vi "Mag_&_Temp_Cntrl.vi"() -> ()   [LabVIEW 2025]
uses:
  CTLS/Status Indicators.ctl
  CTLS/Sweeper.ctl
  CTLS/Scan_Params (QMH).ctl
  CTLS/PSU Status.ctl
  CTLS/TC-Cluster.ctl
  CTLS/ACK.ctl
  <userlib>/Nanonis Prog Interface V5e/Nanonis Prog Interface.lvlib
panel:
  in  "Field and Temp Array Controller":cluster{"Field (T)":dbl[], "Temps (K)":dbl[]}
  out "Status Indicator":T1={"Sweep States"=enum."1. Idle", "PointStep"=enum."1. Scan_1", "Current Field"=0.0, "Current Temp"=0.0, "Expected_ACK"=enum."1. None", "AfterAckStep"=enum."1. Idle", "Current Index Field"=0, "Current Index Temp"=0, "ACK Structure "=enum."Inner"}
  in  "Stop Button":bool
  in  "Stop Experiment":bool
  in  "Start Experiment":bool
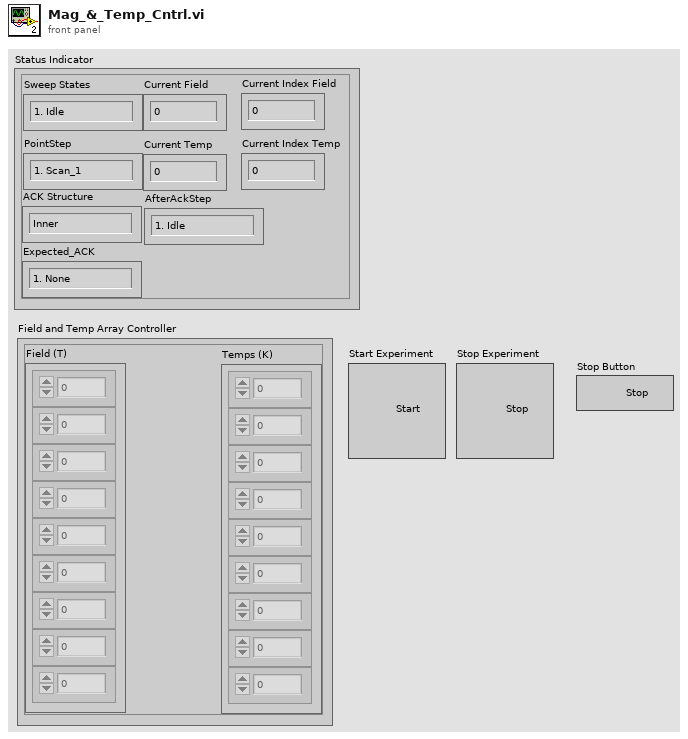
[diagram p1: front panel]
types:
  T1 = typedef "Status Indicators.ctl" = cluster{"Sweep States":enum16{"1. Idle", "2. Start", "3. Apply_Config", "4. Run_Point_Step", "5. Wait ACK", "6. Next Field", "7. Next Temp", "8. Stop"}, "PointStep":enum16{"1. Init_Bias", "2. Init_Scan", "3. Field_Stable", "4. Temp_stable", "1. Scan_1", "2. DC_SF_1", "3. DC_BS_1", "4. Bias", "5. Scan_2", "6. DC_SF_2", "7. DC_BS_2", "8. Done"}, "Current Field":dbl, "Current Temp":dbl, "Expected_ACK":enum16{"1. None", "2. TempStable", "3. FieldStable", "4. ConfigApplied", "5. ScanDone", "6. BiasDone", "7. DriftDone (SF)", "8. DrifDone (BS)", "9. Done"}, "AfterAckStep":enum16{"1. Idle", "2. Start", "3. Apply_Config", "4. Run_Point_Step", "5. Wait ACK", "6. Next Field", "7. Next Temp", "8. Stop"}, "Current Index Field":i32, "Current Index Temp":i32, "ACK Structure ":enum16{"Inner", "Outer"}}
  T2 = enum16{"1. INIT TEMP", "2. TC ON", "3. TEMP_STAB", "4. TC IDLE", "5. TC OFF (Reset)"}
  T3 = typedef "TC-Cluster.ctl" = cluster{"Range (0:Off)":u16, "Manual Output (0.00 %)":dbl, "Rate (D) (0.0 %)":dbl, "Reset (I) (20.0)":dbl, "Gain (P) (50.0)":dbl, "Power Up Enable (F: Disable)":bool, "Max User Current (2.000)":dbl, "Heater Resistance (1:25 Ohms)":u16, "Max Current (0:User Specified)":u16, "Heater Out Display (1:Current)":u16, "Mode (0:Off)":u16, "Input (0:None)":u16, "Target Temp (K)":dbl, "Serial Configuration":cluster{"Baud Rate":u32, "Parity":u16, "Data Bits":u16, "Stop Bits":u16, "Flow Control":u16}, "VISA resource name":refnum<visa-resource-name>, "Configure Control Parameters (0: Configure)":u16, "Enable Setpoint (F:Disable)":bool, "Input (0:A)":u16, "Data Source (0:Kelvin)":u16, "Output's Control Loop (1:1)":u16, "STND DEV Threshold ":dbl, "Mean Tolerance ":dbl, "Current State":enum16{"1. INIT TEMP", "2. TC ON", "3. TEMP_STAB", "4. TC IDLE", "5. TC OFF (Reset)"}}
  T4 = enum16{"1. Idle", "2. Start", "3. Apply_Config", "4. Run_Point_Step", "5. Wait ACK", "6. Next Field", "7. Next Temp", "8. Stop"}
  T5 = typedef "Sweeper.ctl" = cluster{"Temps(K)":dbl[], "Fields(T)":dbl[], "Sweep States":enum16{"1. Idle", "2. Start", "3. Apply_Config", "4. Run_Point_Step", "5. Wait ACK", "6. Next Field", "7. Next Temp", "8. Stop"}, "PointStep":enum16{"1. Init_Bias", "2. Init_Scan", "3. Field_Stable", "4. Temp_stable", "1. Scan_1", "2. DC_SF_1", "3. DC_BS_1", "4. Bias", "5. Scan_2", "6. DC_SF_2", "7. DC_BS_2", "8. Done"}, "Current Field":dbl, "Current Temp":dbl, "Expected_ACK":enum16{"1. None", "2. TempStable", "3. FieldStable", "4. ConfigApplied", "5. ScanDone", "6. BiasDone", "7. DriftDone (SF)", "8. DrifDone (BS)", "9. Done"}, "ACK":enum16{"1. None", "2. TempStable", "3. FieldStable", "4. ConfigApplied", "5. ScanDone", "6. BiasDone", "7. DriftDone (SF)", "8. DrifDone (BS)", "9. Done"}, "AfterAckStep":enum16{"1. Idle", "2. Start", "3. Apply_Config", "4. Run_Point_Step", "5. Wait ACK", "6. Next Field", "7. Next Temp", "8. Stop"}, "Current Index Field":i32, "Current Index Temp":i32, "ACK Structure ":enum16{"Inner", "Outer"}}
  T6 = enum16{"1. INIT MAG", "2. MAG ON", "3. MAG_STAB", "4. MAG IDLE", "5. MAG OFF (Reset)"}
  T7 = typedef "PSU Status.ctl" = cluster{"Ramp Target":enum16{"ZERO", "MID", "MAX"}, "Pause":bool, "Switch Heater":bool, "Persistent Field":dbl, "Persistent Current":dbl, "Tesla":bool, "Output (T)":dbl, "Output (A)":dbl, "X Trip":enum16{"DISABLED", "ENABLED", "ACTIVE"}, "Ramp Rate (A/s)":dbl, "V Limit (V)":dbl, "Heater Voltage":dbl, "MAX Setpoint (A)":dbl, "MAX Setpoint (T)":dbl, "MID Setpoint (A)":dbl, "MID Setpoint (T)":dbl, "Lock":bool, "Field Constant":dbl, "Remote":bool, "Direction":enum16{"POSITIVE", "NEGATIVE", "OPEN", "UNIPOLAR"}, "Helium Level":u16, "Quench !":bool, "Voltage":dbl, "V Limit !":bool, "Ramping":bool, "At Target":bool, "Trip Field":dbl, "Trip Current":dbl, "Current State":enum16{"1. INIT MAG", "2. MAG ON", "3. MAG_STAB", "4. MAG IDLE", "5. MAG OFF (Reset)"}, "MAG Reference":refnum<visa-resource-name>}
  T8 = enum16{"1. BIAS", "2. POLL BIAS", "3. SCAN", "4. SCAN_IDLE", "5. Drift_Correct (SF)", "6. Drift_Correct (BS)", "7. STOP"}
  T9 = typedef "Scan_Params (QMH).ctl" = cluster{"Setpoint (I)":dbl[], "Bias (V)":dbl[], "Number of scans":u8, "Port number (3364)":u32, "Avoid zero threshold (V)":dbl, "Current State":enum16{"1. BIAS", "2. POLL BIAS", "3. SCAN", "4. SCAN_IDLE", "5. Drift_Correct (SF)", "6. Drift_Correct (BS)", "7. STOP"}}
  T10 = typedef "ACK.ctl" = cluster{"ACK":enum16{"1. None", "2. TempStable", "3. FieldStable", "4. ConfigApplied", "5. ScanDone", "6. BiasDone", "7. DriftDone (SF)", "8. DrifDone (BS)"}}
  T11 = enum16{"1. None", "2. TempStable", "3. FieldStable", "4. ConfigApplied", "5. ScanDone", "6. BiasDone", "7. DriftDone (SF)", "8. DrifDone (BS)"}
  T12 = enum16{"1. Init_Bias", "2. Init_Scan", "3. Field_Stable", "4. Temp_stable", "1. Scan_1", "2. DC_SF_1", "3. DC_BS_1", "4. Bias", "5. Scan_2", "6. DC_SF_2", "7. DC_BS_2", "8. Done"}
  T13 = enum16{"1. None", "2. TempStable", "3. FieldStable", "4. ConfigApplied", "5. ScanDone", "6. BiasDone", "7. DriftDone (SF)", "8. DrifDone (BS)", "9. Done"}
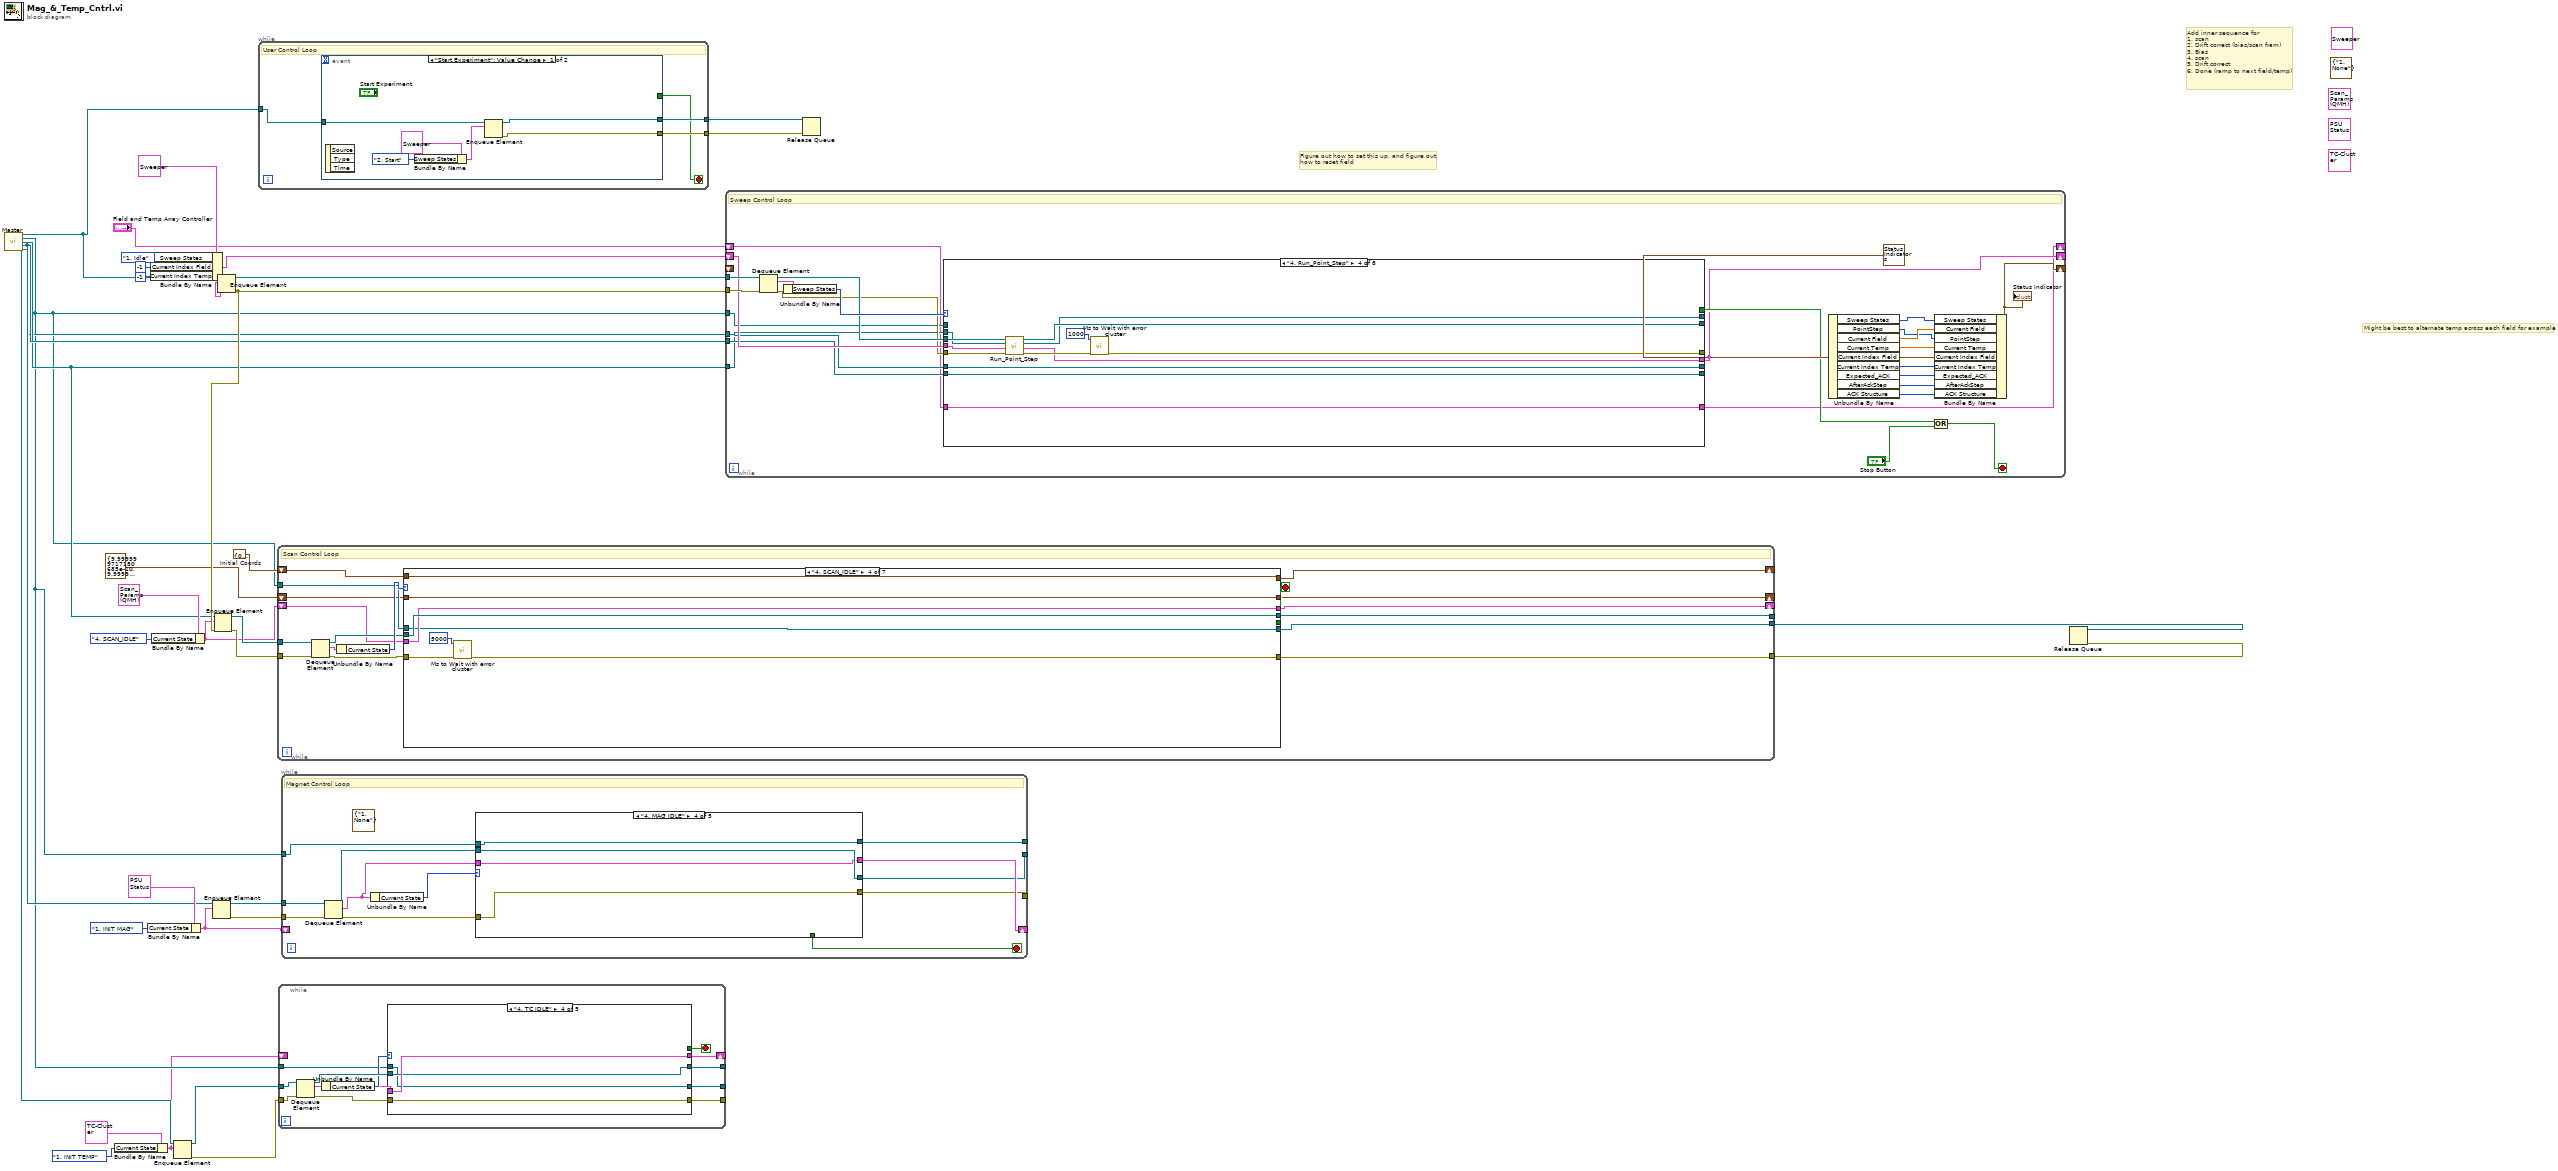
[diagram p0: block diagram]
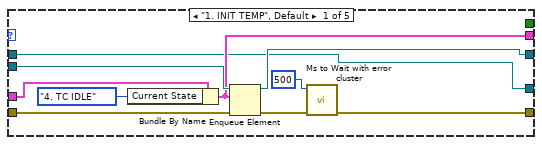
[diagram p2: hidden frame]
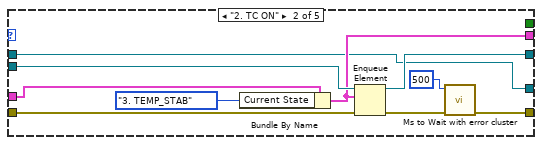
[diagram p3: hidden frame]
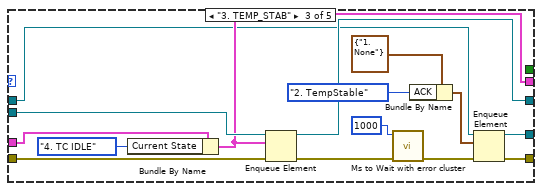
[diagram p4: hidden frame]
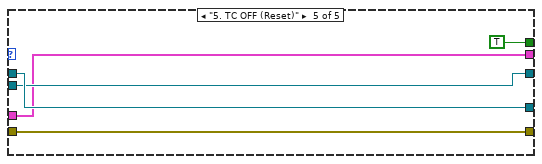
[diagram p5: hidden frame]
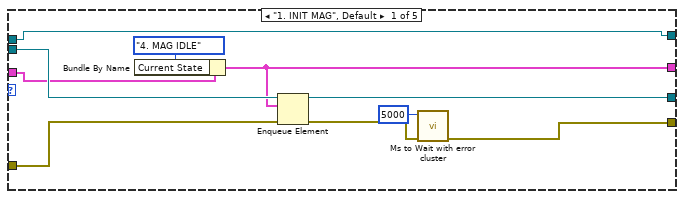
[diagram p6: hidden frame]
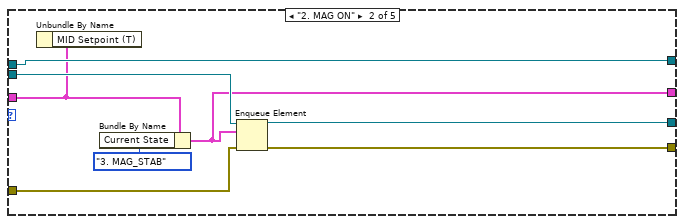
[diagram p7: hidden frame]
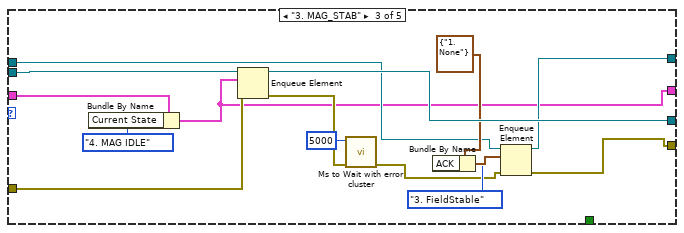
[diagram p8: hidden frame]
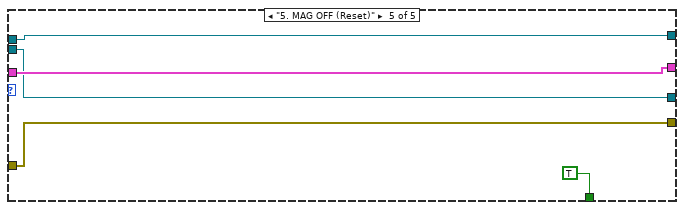
[diagram p9: hidden frame]
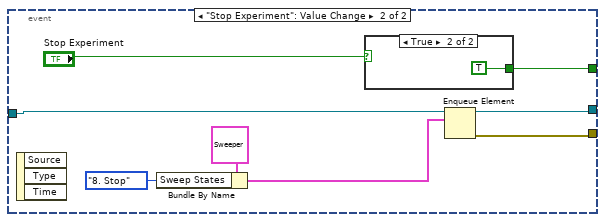
[diagram p10: hidden frame]
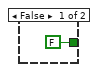
[diagram p11: hidden frame]
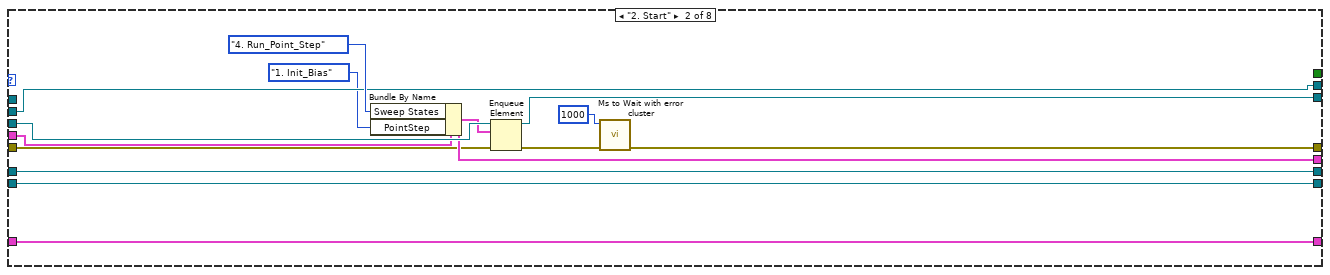
[diagram p13: hidden frame]
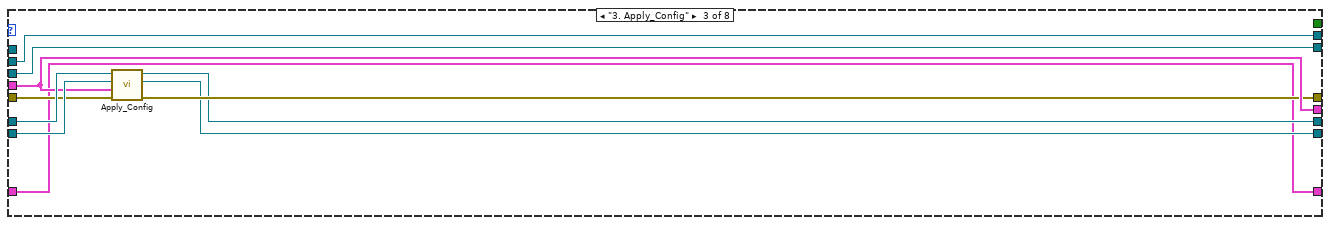
[diagram p14: hidden frame]
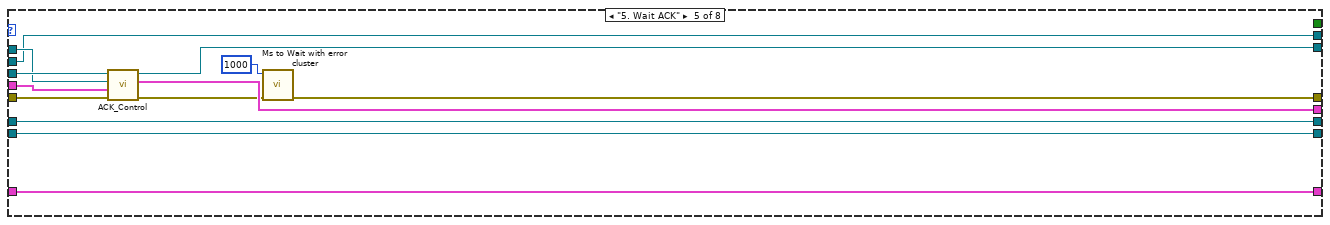
[diagram p15: hidden frame]
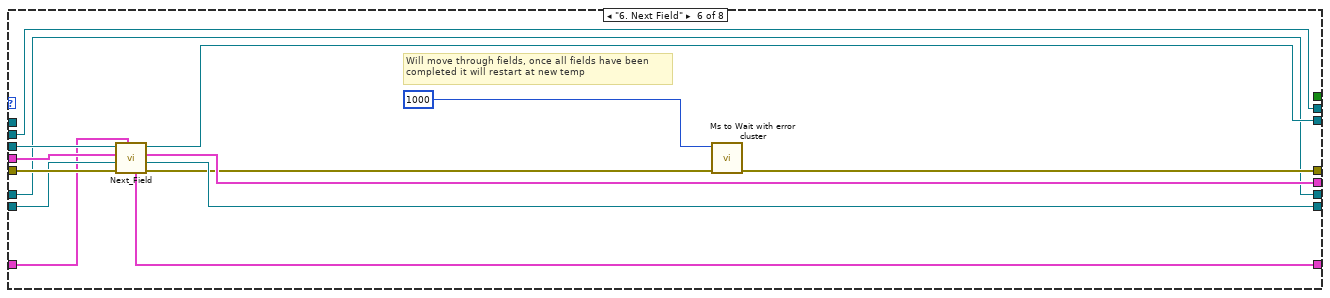
[diagram p16: hidden frame]
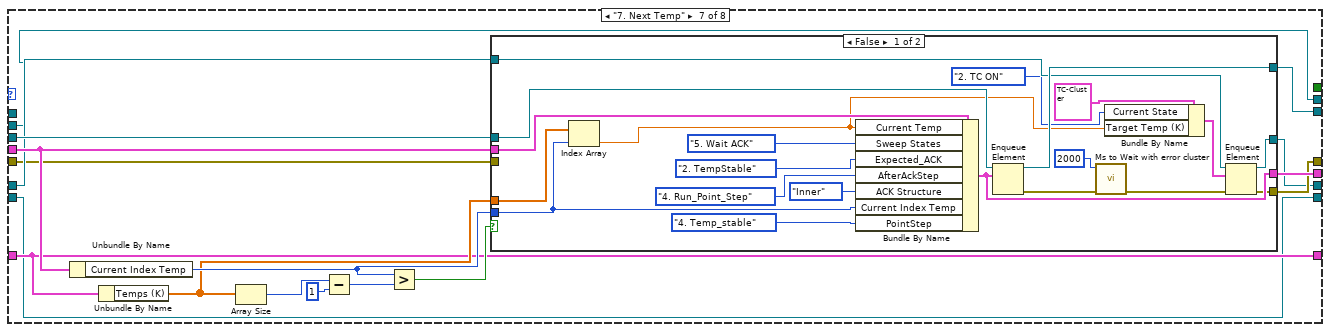
[diagram p17: hidden frame]
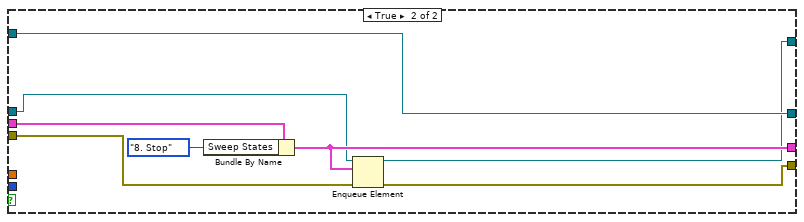
[diagram p18: hidden frame]
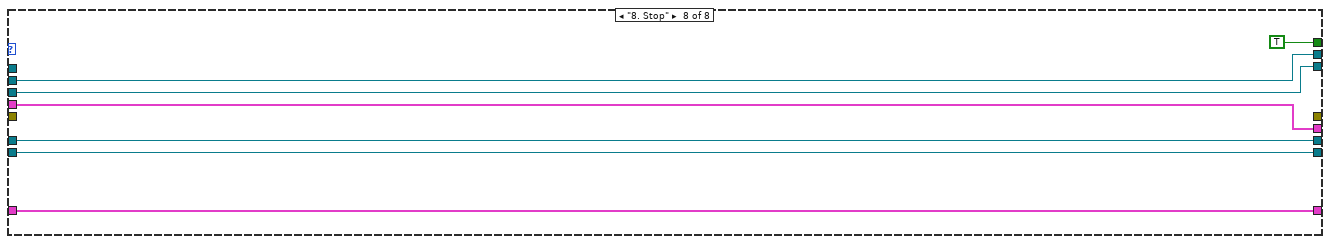
[diagram p19: hidden frame]
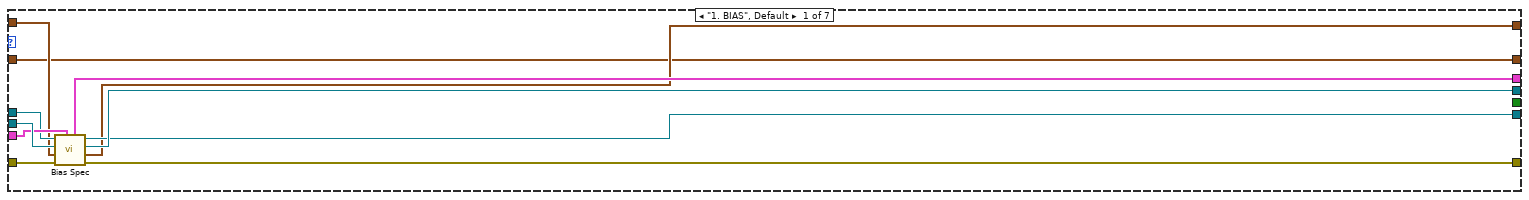
[diagram p20: hidden frame]
diagram:
  w15 = cluster{"Initial x":dbl, "Initial y":dbl} {"Initial x"=0.0, "Initial y"=0.0}  # Initial Coords
  (unwired) T10 {"ACK"=enum."1. None"} ("Acknowledements")
  (unwired) T5 {"Temps(K)"=[], "Fields(T)"=[], "Sweep States"=enum."1. Idle", "PointStep"=enum."1. Scan_1", "Current Field"=0.0, "Current Temp"=0.0, "Expected_ACK"=enum."1. None", "ACK"=enum."1. None", "AfterAckStep"=enum."1. Idle", "Current Index Field"=0, "Current Index Temp"=0, "ACK Structure "=enum."Inner"} ("Temp and Field Range")
  (unwired) T3 {"Range (0:Off)"=0, "Manual Output (0.00 %)"=0.0, "Rate (D) (0.0 %)"=0.0, "Reset (I) (20.0)"=20.0, "Gain (P) (50.0)"=50.0, "Power Up Enable (F: Disable)"=FALSE, "Max User Current (2.000)"=2.0, "Heater Resistance (1:25 Ohms)"=1, "Max Current (0:User Specified)"=0, "Heater Out Display (1:Current)"=1, "Mode (0:Off)"=0, "Input (0:None)"=0, "Target Temp (K)"=0.0, "Serial Configuration"={"Baud Rate"=57600, "Parity"=1, "Data Bits"=7, "Stop Bits"=10, "Flow Control"=0}, "VISA resource name"="", "Configure Control Parameters (0: Configure)"=0, "Enable Setpoint (F:Disable)"=FALSE, "Input (0:A)"=0, "Data Source (0:Kelvin)"=0, "Output's Control Loop (1:1)"=1, "STND DEV Threshold "=0.1, "Mean Tolerance "=0.02, "Current State"=enum."1. INIT TEMP"} ("Temp Controller")
  (unwired) T9 {"Setpoint (I)"=[], "Bias (V)"=[], "Number of scans"=1, "Port number (3364)"=3364, "Avoid zero threshold (V)"=0.004999999888241291, "Current State"=enum."1. BIAS"} ("Scan Parameters")
  (unwired) T7 {"Ramp Target"=enum."ZERO", "Pause"=FALSE, "Switch Heater"=FALSE, "Persistent Field"=0.0, "Persistent Current"=0.0, "Tesla"=FALSE, "Output (T)"=0.0, "Output (A)"=0.0, "X Trip"=enum."DISABLED", "Ramp Rate (A/s)"=0.0, "V Limit (V)"=0.0, "Heater Voltage"=0.0, "MAX Setpoint (A)"=0.0, "MAX Setpoint (T)"=0.0, "MID Setpoint (A)"=0.0, "MID Setpoint (T)"=0.0, "Lock"=FALSE, "Field Constant"=0.0, "Remote"=FALSE, "Direction"=enum."POSITIVE", "Helium Level"=0, "Quench !"=FALSE, "Voltage"=0.0, "V Limit !"=FALSE, "Ramping"=FALSE, "At Target"=FALSE, "Trip Field"=0.0, "Trip Current"=0.0, "Current State"=enum."1. INIT MAG", "MAG Reference"="COM4"} ("PSU Status In")
  # "Figure out how to set this up, and figure out\nhow to reset field"
  # "Might be best to alternate temp across each field for example"
  # "Add inner sequence for \n1. scan\n2. Drift correct (bias/scan fram)\n3. Bias\n4. scan\n5. Drift correct\n6. Done (ramp to next field/temp)"
  n1 = call "Master.vi"() -> ("SweepQ"=w32:refnum<queue>, "ACK Q"=w3:refnum<queue>, "ScanQ"=w12:refnum<queue>, "MagQ"=w13:refnum<queue>, "TempQ"=w8:refnum<queue>)  [unwired: 11 in]
  n2 = Bundle By Name(cluster=T3 {"Range (0:Off)"=0, "Manual Output (0.00 %)"=0.0, "Rate (D) (0.0 %)"=0.0, "Reset (I) (20.0)"=20.0, "Gain (P) (50.0)"=50.0, "Power Up Enable (F: Disable)"=FALSE, "Max User Current (2.000)"=2.0, "Heater Resistance (1:25 Ohms)"=1, "Max Current (0:User Specified)"=0, "Heater Out Display (1:Current)"=1, "Mode (0:Off)"=0, "Input (0:None)"=0, "Target Temp (K)"=0.0, "Serial Configuration"={"Baud Rate"=57600, "Parity"=1, "Data Bits"=7, "Stop Bits"=10, "Flow Control"=0}, "VISA resource name"="", "Configure Control Parameters (0: Configure)"=0, "Enable Setpoint (F:Disable)"=FALSE, "Input (0:A)"=0, "Data Source (0:Kelvin)"=0, "Output's Control Loop (1:1)"=1, "STND DEV Threshold "=0.1, "Mean Tolerance "=0.02, "Current State"=enum."1. INIT TEMP"} ("Temp Controller"), "Current State"=T2."1. INIT TEMP") -> (w2:T3)
  n3 = Bundle By Name(cluster=T7 {"Ramp Target"=enum."ZERO", "Pause"=FALSE, "Switch Heater"=FALSE, "Persistent Field"=0.0, "Persistent Current"=0.0, "Tesla"=FALSE, "Output (T)"=0.0, "Output (A)"=0.0, "X Trip"=enum."DISABLED", "Ramp Rate (A/s)"=0.0, "V Limit (V)"=0.0, "Heater Voltage"=0.0, "MAX Setpoint (A)"=0.0, "MAX Setpoint (T)"=0.0, "MID Setpoint (A)"=0.0, "MID Setpoint (T)"=0.0, "Lock"=FALSE, "Field Constant"=0.0, "Remote"=FALSE, "Direction"=enum."POSITIVE", "Helium Level"=0, "Quench !"=FALSE, "Voltage"=0.0, "V Limit !"=FALSE, "Ramping"=FALSE, "At Target"=FALSE, "Trip Field"=0.0, "Trip Current"=0.0, "Current State"=enum."1. INIT MAG", "MAG Reference"="COM4"} ("PSU Status In"), "Current State"=T6."1. INIT MAG") -> (w19:T7)
  n4 = Bundle By Name(cluster=T5 {"Temps(K)"=[0.0, 1.0], "Fields(T)"=[0.0, 1.0], "Sweep States"=enum."1. Idle", "PointStep"=enum."1. Scan_1", "Current Field"=0.0, "Current Temp"=0.0, "Expected_ACK"=enum."1. None", "ACK"=enum."1. None", "AfterAckStep"=enum."1. Idle", "Current Index Field"=0, "Current Index Temp"=0, "ACK Structure "=enum."Inner"} ("Temp and Field Range"), "Sweep States"=T4."1. Idle", "Current Index Field"=-1, "Current Index Temp"=-1) -> (w14:T5)
  n5 = Bundle By Name(cluster=T9 {"Setpoint (I)"=[], "Bias (V)"=[], "Number of scans"=1, "Port number (3364)"=3364, "Avoid zero threshold (V)"=0.004999999888241291, "Current State"=enum."1. BIAS"} ("Scan Parameters"), "Current State"=T8."4. SCAN_IDLE") -> (w24:T9)
  n6 = Enqueue Element(queue=w8, element=w2) -> (queue out=w5:refnum<queue>, error out=w4:errorcluster)  [unwired: 2 in, 1 out]
  n7 = Enqueue Element(queue=w13, element=w19) -> (queue out=w23:refnum<queue>, error out=w22:errorcluster)  [unwired: 2 in, 1 out]
  n8 = Enqueue Element(queue=w32, element=w14) -> (queue out=w34:refnum<queue>, error out=w27:errorcluster)  [unwired: 2 in, 1 out]
  n9 = Enqueue Element(queue=w12, element=w24, error in (no error)=w27) -> (queue out=w33:refnum<queue>, error out=w28:errorcluster)  [unwired: 1 in, 1 out]
  n10 = while {
    tunnel: w32 -> [w38]
    tunnel: [w37] -> w31
    tunnel: [w36] -> w30
    stop <- w35 stop-if-true
    # "User Control Loop"
    n11 = event shown="[0] \"Start Experiment\": Value Change" {
      selector: _ -> [_ _]
      dyn-events: _ -> [_ _]
      timeout: _ -> [_ _]
      tunnel: w38 -> [w44 w52]
      tunnel: [w41 w49] -> w37
      tunnel: [w40 w48] -> w36
      tunnel: [_ w46] -> w35
      event "Start Experiment": Value Change {
        n12 = event-data() -> ()  [unwired: 1 in, 3 out]
        n13 = Bundle By Name(cluster=T5 {"Temps(K)"=[], "Fields(T)"=[], "Sweep States"=enum."1. Idle", "PointStep"=enum."1. Scan_1", "Current Field"=0.0, "Current Temp"=0.0, "Expected_ACK"=enum."1. None", "ACK"=enum."1. None", "AfterAckStep"=enum."1. Idle", "Current Index Field"=0, "Current Index Temp"=0, "ACK Structure "=enum."Inner"} ("Temp and Field Range"), "Sweep States"=T4."2. Start") -> (w42:T5)
        n14 = Enqueue Element(queue=w44, element=w42) -> (queue out=w41:refnum<queue>, error out=w40:errorcluster)  [unwired: 2 in, 1 out]
      }
      event "Stop Experiment": Value Change {
        n15 = event-data() -> ()  [unwired: 1 in, 3 out]
        n16 = Bundle By Name(cluster=T5 {"Temps(K)"=[], "Fields(T)"=[], "Sweep States"=enum."1. Idle", "PointStep"=enum."1. Scan_1", "Current Field"=0.0, "Current Temp"=0.0, "Expected_ACK"=enum."1. None", "ACK"=enum."1. None", "AfterAckStep"=enum."1. Idle", "Current Index Field"=0, "Current Index Temp"=0, "ACK Structure "=enum."Inner"} ("Temp and Field Range"), "Sweep States"=T4."8. Stop") -> (w50:T5)
        n17 = case shown="True" "Stop Experiment" {
          tunnel: [FALSE TRUE] -> w46
          frame False {
          }
          frame True {
          }
        }
        n18 = Enqueue Element(queue=w52, element=w50) -> (queue out=w49:refnum<queue>, error out=w48:errorcluster)  [unwired: 2 in, 1 out]
      }
    }
  }
  n19 = while {
    tunnel: w3 -> [w63]
    tunnel: w33 -> [w71]
    tunnel: w28 -> [w68]
    shift-right: [w60] -> _
    shift-left: w24 -> [w61]
    tunnel: [w66] -> _
    tunnel: [w64] -> w9
    tunnel: [w62] -> w10
    shift-right: [w57] -> _
    shift-left: w15 -> [w58]
    shift-right: [w55] -> _
    shift-left: cluster{"Dx":sgl, "Dy":sgl} {"Dx"=1e-09, "Dy"=1e-09} ("Dx, Dy") -> [w56]
    stop <- w59 stop-if-true
    # "Scan Control Loop"
    n20 = Dequeue Element(queue=w71, error in (no error)=w68) -> (queue out=w67:refnum<queue>, element=w70:T9, error out=w65:errorcluster)  [unwired: 1 in, 1 out]
    n21 = Unbundle By Name(w70) -> ("Current State"=w69:T8)
    n22 = case shown="\"4. SCAN_IDLE\"" w69 {
      tunnel: w67 -> [w82 w92 w102 w118 w126 w144 w162]
      tunnel: [w81 w91 w105 w118 w127 w146 w163] -> w66
      tunnel: w65 -> [w73 w90 _ w113 _ w143 _]
      tunnel: [w76 w85 w97 w116 w122 w138 w156] -> w64
      tunnel: w63 -> [w77 w89 w103 w114 w125 w145 w161]
      tunnel: [w78 w88 w104 w114 w128 w147 w164] -> w62
      tunnel: [w79 w86 w100 w117 w123 w140 w159] -> w60
      tunnel: w61 -> [w80 w87 w101 w117 w124 w141 w160]
      tunnel: [_ _ _ _ _ _ TRUE] -> w59
      tunnel: w58 -> [w75 w84 w94 w112 w119 w133 w153]
      tunnel: [w74 w84 w94 w112 w119 w130 w153] -> w57
      tunnel: w56 -> [w72 w83 w93 w111 w121 w136 w152]
      tunnel: [w72 w83 w93 w111 w120 w136 w152] -> w55
      frame "1. BIAS", Default {
        n23 = call "Bias Spec.vi"("Scan Parameters in"=w80, "error in (no error)"=w73, "Cluster"=w75, "ScanQ in"=w82, "Queue in"=w77) -> ("error out"=w76:errorcluster, "output cluster"=w74:cluster{"Initial x":dbl, "Initial y":dbl}, "ScanQ out"=w81:refnum<queue>, "Queue out"=w78:refnum<queue>, "Scan Parameters out"=w79:T9)  [unwired: 2 in]
      }
      frame "2. POLL BIAS" {
        n24 = call "Poll_Bias.vi"("error in (no error)"=w90, "Scan Parameters in"=w87, "ACK Q in"=w89, "Queue in"=w92) -> ("error out"=w85:errorcluster, "Scan Parameters out"=w86:T9, "ACK Q out"=w88:refnum<queue>, "Queue out"=w91:refnum<queue>)  [unwired: 4 in]
      }
      frame "3. SCAN" {
        n25 = Bundle By Name(cluster=w101, "Current State"=T8."4. SCAN_IDLE") -> (w100:T9)
        n26 = call "Scan Multi Bias (With Setpoint Control-REVISED).vi"("Number of scans"=u8 1) -> ("Error out"=w95:errorcluster)  [unwired: 14 in]
        n27 = Bundle By Name(cluster=T10 {"ACK"=enum."1. None"} ("Acknowledements"), "ACK"=T11."5. ScanDone") -> (w108:T10)
        n28 = Enqueue Element(queue=w102, element=w100, error in (no error)=w95) -> (queue out=w105:refnum<queue>, error out=w107:errorcluster)  [unwired: 1 in, 1 out]
        n29 = Enqueue Element(queue=w103, element=w108, error in (no error)=w107) -> (queue out=w104:refnum<queue>, error out=w98:errorcluster)  [unwired: 1 in, 1 out]
        n30 = call <userlib>:"Ms to Wait with error cluster.vi"("error in (no error)"=w98, "milliseconds to wait"=u32 5000) -> ("error out"=w97:errorcluster)  [unwired: 4 in, 1 out]
      }
      frame "4. SCAN_IDLE" {
        n31 = call <userlib>:"Ms to Wait with error cluster.vi"("error in (no error)"=w113, "milliseconds to wait"=u32 5000) -> ("error out"=w116:errorcluster)  [unwired: 4 in, 1 out]
      }
      frame "5. Drift_Correct (SF)" {
        n32 = call "Drift Correct Scan Frame.vi"("Scan Parameters in"=w124, "ScanQ in"=w126, "Dx, Dy"=w121, "Queue in"=w125) -> ("error out"=w122:errorcluster, "Dx, Dy 2"=w120:cluster{"Dx":sgl, "Dy":sgl}, "Scan Parameters out"=w123:T9, "Queue out"=w128:refnum<queue>, "ScanQ out"=w127:refnum<queue>)  [unwired: 2 in, 1 out]
      }
      frame "6. Drift_Correct (BS)" {
        # "Need to add Bias Shift"
        n33 = Unbundle By Name(w133) -> ("Initial x"=w135:dbl, "Initial y"=w134:dbl)
        n34 = call "MOVE BIAS.vi"("Dx, Dy"=w136, "Initial X"=w135, "Boolean"=TRUE, "Initial Y"=w134) -> ("FInal X (m)"=w132:sgl, "Final Y (m)"=w131:sgl)  [unwired: 10 in]
        n35 = Bundle By Name(cluster=w133, "Initial x"=w132, "Initial y"=w131) -> (w130:cluster{"Initial x":dbl, "Initial y":dbl})
        n36 = Bundle By Name(cluster=w141, "Current State"=T8."4. SCAN_IDLE") -> (w140:T9)
        n37 = Bundle By Name(cluster=T10 {"ACK"=enum."1. None"} ("Acknowledements"), "ACK"=T11."8. DrifDone (BS)") -> (w150:T10)
        n38 = Enqueue Element(queue=w144, element=w140, error in (no error)=w143) -> (queue out=w146:refnum<queue>, error out=w149:errorcluster)  [unwired: 1 in, 1 out]
        n39 = Enqueue Element(queue=w145, element=w150, error in (no error)=w149) -> (queue out=w147:refnum<queue>, error out=w139:errorcluster)  [unwired: 1 in, 1 out]
        n40 = call <userlib>:"Ms to Wait with error cluster.vi"("error in (no error)"=w139, "milliseconds to wait"=u32 5000) -> ("error out"=w138:errorcluster)  [unwired: 4 in, 1 out]
      }
      frame "7. STOP" {
        n41 = Bundle By Name(cluster=w160, "Current State"=T8."4. SCAN_IDLE") -> (w159:T9)
        n42 = Bundle By Name(cluster=T10 {"ACK"=enum."1. None"} ("Acknowledements"), "ACK"=T11."1. None") -> (w167:T10)
        n43 = Enqueue Element(queue=w162, element=w159) -> (queue out=w163:refnum<queue>, error out=w166:errorcluster)  [unwired: 2 in, 1 out]
        n44 = Enqueue Element(queue=w161, element=w167, error in (no error)=w166) -> (queue out=w164:refnum<queue>, error out=w157:errorcluster)  [unwired: 1 in, 1 out]
        n45 = call <userlib>:"Ms to Wait with error cluster.vi"("error in (no error)"=w157, "milliseconds to wait"=u32 5000) -> ("error out"=w156:errorcluster)  [unwired: 4 in, 1 out]
      }
    }
  }
  n46 = while {
    tunnel: w5 -> [w180]
    tunnel: w4 -> [w179]
    tunnel: w3 -> [w171]
    tunnel: [w175] -> _
    tunnel: [w173] -> _
    shift-right: [w172] -> _
    shift-left: w2 -> [_]
    tunnel: [w170] -> _
    stop <- w169 stop-if-true
    n47 = Dequeue Element(queue=w180, error in (no error)=w179) -> (queue out=w178:refnum<queue>, element=w176:T3, error out=w174:errorcluster)  [unwired: 1 in, 1 out]
    n48 = Unbundle By Name(w176) -> ("Current State"=w177:T2)
    n49 = case shown="\"4. TC IDLE\"" w177 {
      tunnel: w178 -> [w190 w198 w213 w218 w221]
      tunnel: w176 -> [w189 w200 w215 w219 w220]
      tunnel: [w187 w193 w207 w218 w221] -> w175
      tunnel: w174 -> [w186 w197 w212 w216 w223]
      tunnel: [w184 w194 w208 w216 w223] -> w173
      tunnel: [w185 w192 w206 w219 w220] -> w172
      tunnel: w171 -> [w181 w191 w205 w217 w222]
      tunnel: [w181 w191 w201 w217 w222] -> w170
      tunnel: [_ _ _ _ TRUE] -> w169
      frame "1. INIT TEMP", Default {
        n50 = Bundle By Name(cluster=w189, "Current State"=T2."4. TC IDLE") -> (w185:T3)
        n51 = Enqueue Element(queue=w190, element=w185, error in (no error)=w186) -> (queue out=w187:refnum<queue>, error out=w183:errorcluster)  [unwired: 1 in, 1 out]
        n52 = call <userlib>:"Ms to Wait with error cluster.vi"("error in (no error)"=w183, "milliseconds to wait"=u32 500) -> ("error out"=w184:errorcluster)  [unwired: 4 in, 1 out]
      }
      frame "2. TC ON" {
        n53 = Bundle By Name(cluster=w200, "Current State"=T2."3. TEMP_STAB") -> (w192:T3)
        n54 = Enqueue Element(queue=w198, element=w192, error in (no error)=w197) -> (queue out=w193:refnum<queue>, error out=w195:errorcluster)  [unwired: 1 in, 1 out]
        n55 = call <userlib>:"Ms to Wait with error cluster.vi"("error in (no error)"=w195, "milliseconds to wait"=u32 500) -> ("error out"=w194:errorcluster)  [unwired: 4 in, 1 out]
      }
      frame "3. TEMP_STAB" {
        n56 = Bundle By Name(cluster=w215, "Current State"=T2."4. TC IDLE") -> (w206:T3)
        n57 = Enqueue Element(queue=w213, element=w206, error in (no error)=w212) -> (queue out=w207:refnum<queue>, error out=w211:errorcluster)  [unwired: 1 in, 1 out]
        n58 = call <userlib>:"Ms to Wait with error cluster.vi"("error in (no error)"=w211, "milliseconds to wait"=u32 1000) -> ("error out"=w209:errorcluster)  [unwired: 4 in, 1 out]
        n59 = Bundle By Name(cluster=T10 {"ACK"=enum."1. None"} ("Acknowledements"), "ACK"=T11."2. TempStable") -> (w202:T10)
        n60 = Enqueue Element(queue=w205, element=w202, error in (no error)=w209) -> (queue out=w201:refnum<queue>, error out=w208:errorcluster)  [unwired: 1 in, 1 out]
      }
      frame "4. TC IDLE" {
      }
      frame "5. TC OFF (Reset)" {
      }
    }
  }
  n61 = while {
    tunnel: w3 -> [w227]
    tunnel: w23 -> [w236]
    tunnel: w22 -> [w235]
    shift-right: [w230] -> _
    shift-left: w19 -> [_]
    tunnel: [w229] -> _
    tunnel: [w228] -> _
    tunnel: [w226] -> _
    stop <- w225 stop-if-true
    (unwired) T10 {"ACK"=enum."1. None"} ("Acknowledements")
    # "Magnet Control Loop"
    n62 = Dequeue Element(queue=w236, error in (no error)=w235) -> (queue out=w233:refnum<queue>, element=w231:T7, error out=w232:errorcluster)  [unwired: 1 in, 1 out]
    n63 = Unbundle By Name(w231) -> ("Current State"=w234:T6)
    n64 = case shown="\"4. MAG IDLE\"" w234 {
      tunnel: w233 -> [w245 w254 w268 w272 w276]
      tunnel: w232 -> [w246 w253 w269 w273 w275]
      tunnel: w231 -> [w244 w247 w267 w270 w277]
      tunnel: [w242 w249 w255 w270 w277] -> w230
      tunnel: [w241 w251 w263 w272 w276] -> w229
      tunnel: [w239 w250 w257 w273 w275] -> w228
      tunnel: w227 -> [w237 w248 w259 w271 w278]
      tunnel: [w237 w248 w258 w271 w278] -> w226
      tunnel: [_ _ _ _ TRUE] -> w225
      frame "1. INIT MAG", Default {
        n65 = Bundle By Name(cluster=w244, "Current State"=T6."4. MAG IDLE") -> (w242:T7)
        n66 = Enqueue Element(queue=w245, element=w242, error in (no error)=w246) -> (queue out=w241:refnum<queue>, error out=w240:errorcluster)  [unwired: 1 in, 1 out]
        n67 = call <userlib>:"Ms to Wait with error cluster.vi"("error in (no error)"=w240, "milliseconds to wait"=u32 5000) -> ("error out"=w239:errorcluster)  [unwired: 4 in, 1 out]
      }
      frame "2. MAG ON" {
        n68 = Unbundle By Name(w247) -> ()  [unwired: 1 out]
        n69 = Bundle By Name(cluster=w247, "Current State"=T6."3. MAG_STAB") -> (w249:T7)
        n70 = Enqueue Element(queue=w254, element=w249, error in (no error)=w253) -> (queue out=w251:refnum<queue>, error out=w250:errorcluster)  [unwired: 1 in, 1 out]
      }
      frame "3. MAG_STAB" {
        n71 = Bundle By Name(cluster=w267, "Current State"=T6."4. MAG IDLE") -> (w255:T7)
        n72 = Enqueue Element(queue=w268, element=w255, error in (no error)=w269) -> (queue out=w263:refnum<queue>, error out=w265:errorcluster)  [unwired: 1 in, 1 out]
        n73 = call <userlib>:"Ms to Wait with error cluster.vi"("error in (no error)"=w265, "milliseconds to wait"=u32 5000) -> ("error out"=w256:errorcluster)  [unwired: 4 in, 1 out]
        n74 = Bundle By Name(cluster=T10 {"ACK"=enum."1. None"} ("Acknowledements"), "ACK"=T11."3. FieldStable") -> (w261:T10)
        n75 = Enqueue Element(queue=w259, element=w261, error in (no error)=w256) -> (queue out=w258:refnum<queue>, error out=w257:errorcluster)  [unwired: 1 in, 1 out]
      }
      frame "4. MAG IDLE" {
      }
      frame "5. MAG OFF (Reset)" {
      }
    }
  }
  n76 = while {
    tunnel: w34 -> [w306]
    tunnel: w27 -> [w304]
    shift-right: [w282] -> _
    shift-left: _ -> [_]
    tunnel: w3 -> [w288]
    tunnel: w13 -> [w287]
    tunnel: w8 -> [w286]
    tunnel: w12 -> [w285]
    shift-right: [w281] -> _
    shift-left: w14 -> [w290]
    shift-right: [w280] -> _
    shift-left: "Field and Temp Array Controller" -> [w284]
    stop <- w302 stop-if-true
    # "Sweep Control Loop"
    n77 = Dequeue Element(queue=w306, error in (no error)=w304) -> (queue out=w291:refnum<queue>, element=w305:T5, error out=w289:errorcluster)  [unwired: 1 in, 1 out]
    n78 = Unbundle By Name(w305) -> ("Sweep States"=w292:T4)
    n79 = case shown="\"4. Run_Point_Step\"" w292 {
      tunnel: w291 -> [w308 w326 w329 w345 w362 w374 w384 w425]
      tunnel: w290 -> [w312 w325 w334 w343 w360 w376 w389 w428]
      tunnel: [w312 w324 w334 w342 w357 w375 w388 w428] -> w281
      tunnel: [w308 w323 w329 w341 w358 w373 w383 w425] -> _
      tunnel: w289 -> [_ w322 w333 w349 w359 w372 w379 _]
      tunnel: [_ w319 w332 w347 w355 w367 w381 _] -> _
      tunnel: w288 -> [_ _ _ _ w361 _ _ _]
      tunnel: w287 -> [w309 w315 w336 w339 w351 w370 w377 w426]
      tunnel: w286 -> [w311 w316 w335 w338 w352 w365 w382 w424]
      tunnel: w285 -> [w310 w317 w328 w344 w353 w364 w378 w427]
      tunnel: [w309 w315 w331 w339 w351 w371 w377 w426] -> _
      tunnel: [_ _ _ _ _ _ _ TRUE ("x")] -> w283
      tunnel: [w311 w316 w330 w338 w352 w365 w380 w424] -> _
      tunnel: [w310 w317 w328 w340 w353 w364 w378 w427] -> _
      tunnel: w284 -> [w307 w314 w327 w337 w350 w369 w385 w423]
      tunnel: [w307 w314 w327 w337 w350 w363 w385 w423] -> w280
      frame "1. Idle" {
      }
      frame "2. Start" {
        n80 = Bundle By Name(cluster=w325, "Sweep States"=T4."4. Run_Point_Step", "PointStep"=T12."1. Init_Bias") -> (w324:T5)
        n81 = Enqueue Element(queue=w326, element=w324, error in (no error)=w322) -> (queue out=w323:refnum<queue>, error out=w321:errorcluster)  [unwired: 1 in, 1 out]
        n82 = call <userlib>:"Ms to Wait with error cluster.vi"("error in (no error)"=w321, "milliseconds to wait"=u32 1000) -> ("error out"=w319:errorcluster)  [unwired: 4 in, 1 out]
      }
      frame "3. Apply_Config" {
        n83 = call "Apply_Config.vi"("error in (no error)"=w333, "Temp and Field Range"=w334, "MagQ"=w336, "Queue in"=w335) -> ("error out"=w332:errorcluster, "MaqQ Our"=w331:refnum<queue>, "TempQ Out"=w330:refnum<queue>)  [unwired: 5 in]
      }
      frame "4. Run_Point_Step" {
        n84 = call "Run_Point_Step.vi"("error in (no error)"=w349, "Producer In"=w343, "ScanQ In"=w344, "SweepQ In"=w345) -> ("error out"=w348:errorcluster, "Producer Out"=w342:T5, "ScanQ Out"=w340:refnum<queue>, "SweepQ Out"=w341:refnum<queue>)  [unwired: 4 in]
        n85 = call <userlib>:"Ms to Wait with error cluster.vi"("error in (no error)"=w348, "milliseconds to wait"=u32 1000) -> ("error out"=w347:errorcluster)  [unwired: 4 in, 1 out]
      }
      frame "5. Wait ACK" {
        n86 = call "ACK_Control.vi"("error in (no error)"=w359, "Producer In"=w360, "ACK Q"=w361, "Queue in"=w362) -> ("error out"=w356:errorcluster, "Producer out"=w357:T5, "Queue out"=w358:refnum<queue>)  [unwired: 5 in]
        n87 = call <userlib>:"Ms to Wait with error cluster.vi"("error in (no error)"=w356, "milliseconds to wait"=u32 1000) -> ("error out"=w355:errorcluster)  [unwired: 4 in, 1 out]
      }
      frame "6. Next Field" {
        # "Will move through fields, once all fields have been\ncompleted it will restart at new temp"
        n88 = call "Next_Field.vi"("Field and Temp Array Controller"=w369, "error in (no error)"=w372, "MagQ In"=w370, "Temp and Field Range in"=w376, "Queue in"=w374) -> ("error out"=w368:errorcluster, "MagQ Out"=w371:refnum<queue>, "Temp and Field Range out"=w375:T5, "Queue out"=w373:refnum<queue>, "Field and Temp Array Controller 3"=w363:cluster{"Field (T)":dbl[], "Temps (K)":dbl[]})  [unwired: 1 in, 1 out]
        n89 = call <userlib>:"Ms to Wait with error cluster.vi"("error in (no error)"=w368, "milliseconds to wait"=u32 1000) -> ("error out"=w367:errorcluster)  [unwired: 4 in, 1 out]
      }
      frame "7. Next Temp" {
        n90 = Unbundle By Name(w389) -> ("Current Index Temp"=w387:i32)
        n91 = Unbundle By Name(w385) -> ("Temps (K)"=w386:dbl[])
        n92 = Array Size(array=w386) -> (size(s)=w392:i32)
        n93 = Subtract(x=w392, y=1 ("x")) -> (x-y=w391:i32)
        n94 = Greater?(x=w387, y=w391) -> (0:w390:bool)
        n95 = case shown="False" w390 {
          tunnel: w389 -> [w414 w422]
          tunnel: w387 -> [w408 _]
          tunnel: [w406 w420] -> w388
          tunnel: w386 -> [w409 _]
          tunnel: w384 -> [w405 w418]
          tunnel: [w404 w417] -> w383
          tunnel: w382 -> [w400 w419]
          tunnel: [w395 w416] -> w381
          tunnel: [w394 w419] -> w380
          tunnel: w379 -> [_ w415]
          frame False {
            n96 = Index Array(array=w409, index=w408) -> (element=w396:dbl)
            n97 = Bundle By Name(cluster=w414, "Current Temp"=w396, "Sweep States"=T4."5. Wait ACK", "Expected_ACK"=T13."2. TempStable", "AfterAckStep"=T4."4. Run_Point_Step", "ACK Structure"=enum16{"Inner", "Outer"}."Inner", "Current Index Temp"=w408, "PointStep"=T12."4. Temp_stable") -> (w406:T5)
            n98 = Enqueue Element(queue=w405, element=w406) -> (queue out=w404:refnum<queue>, error out=w403:errorcluster)  [unwired: 2 in, 1 out]
            n99 = call <userlib>:"Ms to Wait with error cluster.vi"("error in (no error)"=w403, "milliseconds to wait"=u32 2000) -> ("error out"=w401:errorcluster)  [unwired: 4 in, 1 out]
            n100 = Bundle By Name(cluster=T3 {"Range (0:Off)"=0, "Manual Output (0.00 %)"=0.0, "Rate (D) (0.0 %)"=0.0, "Reset (I) (20.0)"=20.0, "Gain (P) (50.0)"=50.0, "Power Up Enable (F: Disable)"=FALSE, "Max User Current (2.000)"=2.0, "Heater Resistance (1:25 Ohms)"=1, "Max Current (0:User Specified)"=0, "Heater Out Display (1:Current)"=1, "Mode (0:Off)"=0, "Input (0:None)"=0, "Target Temp (K)"=0.0, "Serial Configuration"={"Baud Rate"=57600, "Parity"=1, "Data Bits"=7, "Stop Bits"=10, "Flow Control"=0}, "VISA resource name"="", "Configure Control Parameters (0: Configure)"=0, "Enable Setpoint (F:Disable)"=FALSE, "Input (0:A)"=0, "Data Source (0:Kelvin)"=0, "Output's Control Loop (1:1)"=1, "STND DEV Threshold "=0.1, "Mean Tolerance "=0.02, "Current State"=enum."1. INIT TEMP"} ("Temp Controller"), "Current State"=T2."2. TC ON", "Target Temp (K)"=w396) -> (w398:T3)
            n101 = Enqueue Element(queue=w400, element=w398, error in (no error)=w401) -> (queue out=w394:refnum<queue>, error out=w395:errorcluster)  [unwired: 1 in, 1 out]
          }
          frame True {
            n102 = Bundle By Name(cluster=w422, "Sweep States"=T4."8. Stop") -> (w420:T5)
            n103 = Enqueue Element(queue=w418, element=w420, error in (no error)=w415) -> (queue out=w417:refnum<queue>, error out=w416:errorcluster)  [unwired: 1 in, 1 out]
          }
        }
      }
      frame "8. Stop" {
      }
    }
    n104 = Unbundle By Name(w281) -> ("Sweep States"=w294:T4, "PointStep"=w279:T12, "Current Field"=w300:dbl, "Current Temp"=w299:dbl, "Current Index Field"=w295:i32, "Current Index Temp"=w296:i32, "Expected_ACK"=w297:T13, "AfterAckStep"=w293:T4, "ACK Structure"=w298:enum16{"Inner", "Outer"})
    n105 = Or(x=w283, y="Stop Button") -> (x .or. y?=w302:bool)
    n106 = Bundle By Name(cluster=T1 {"Sweep States"=enum."1. Idle", "PointStep"=enum."1. Scan_1", "Current Field"=0.0, "Current Temp"=0.0, "Expected_ACK"=enum."1. None", "AfterAckStep"=enum."1. Idle", "Current Index Field"=0, "Current Index Temp"=0, "ACK Structure "=enum."Inner"} ("Status Indicators"), "Sweep States"=w294, "Current Field"=w300, "PointStep"=w279, "Current Temp"=w299, "Current Index Field"=w295, "Current Index Temp"=w296, "Expected_ACK"=w297, "AfterAckStep"=w293, "ACK Structure"=w298) -> (w282:T1)
    "Status Indicator" <- w282
  }
  n107 = Release Queue(queue=w31, error in (no error)=w30) -> ()  [unwired: 1 in, 3 out]
  n108 = Release Queue(queue=w10, error in (no error)=w9) -> ()  [unwired: 1 in, 3 out]
